vi "Read Field Specs.vi"(8 "error in (no error)":errorcluster, 11 "PitchMessage in":refnum<class "PitchMessage.lvclass">) -> (0 "error out":errorcluster, 2 "Field Specs":T1[](array[typedef])=[{"Name"="Length", "Offset"=0, "Length"=1, "FieldType"=enum."Binary", "FieldValue"=variant}, {"Name"="MessageType", "Offset"=1, "Length"=1, "FieldType"=enum."Value", "FieldValue"=variant}, {"Name"="Time Offset", "Offset"=2, "Length"=4, "FieldType"=enum."Binary", "FieldValue"=variant}, {"Name"="Order Id", "Offset"=6, "Length"=8, "FieldType"=enum."Binary", "FieldValue"=variant}, {"Name"="Side Indicator", "Offset"=14, "Length"=1, "FieldType"=enum."Alphanumeric", "FieldValue"=variant}, {"Name"="Quantity", "Offset"=15, "Length"=4, "FieldType"=enum."Binary", "FieldValue"=variant}, {"Name"="Symbol", "Offset"=19, "Length"=6, "FieldType"=enum."PrintableAscii", "FieldValue"=variant}, {"Name"="Price", "Offset"=25, "Length"=8, "FieldType"=enum."BinaryLongPrice", "FieldValue"=variant}, {"Name"="Add Flags", "Offset"=33, "Length"=1, "FieldType"=enum."BitField", "FieldValue"=variant}], 3 "PitchMessage out":refnum<class "PitchMessage.lvclass">)   [LabVIEW 2020, in "PitchMessage.lvclass"]
uses:
  PitchMessage.lvclass
  FieldSpec.ctl
  PitchMessage.lvclass/PitchMessage.ctl
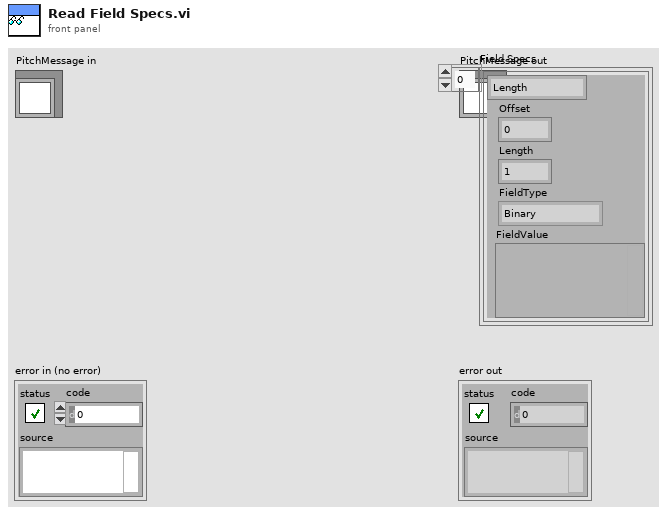
[diagram p1: front panel]
types:
  T1 = typedef "FieldSpec.ctl" = cluster{"Name":string, "Offset":i32, "Length":i32, "FieldType":enum16{"Alphanumeric", "Binary", "BinaryLongPrice", "BinaryShortPrice", "BitField", "PrintableAscii", "Value"}, "FieldValue":variant}
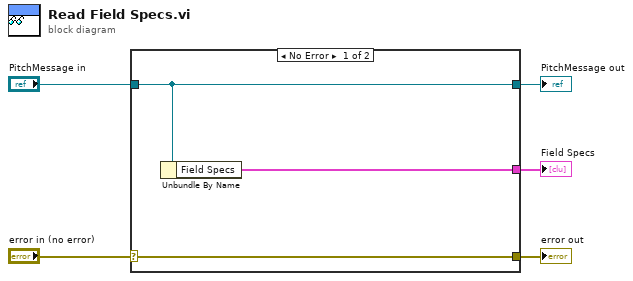
[diagram p0: block diagram]
diagram:
  n1 = case shown="No Error" "error in (no error)" {
    selector: "error in (no error)" -> [w8 w9]
    tunnel: [w8 w9] -> w4
    tunnel: [w7 w10] -> w2
    tunnel: "PitchMessage in" -> [w7 w10]
    tunnel: [w6 _] -> w1
    frame No Error {
      n2 = Unbundle By Name(w7) -> ("Field Specs"=w6:T1[])
    }
    frame Error {
    }
  }
  "error out" <- w4
  "PitchMessage out" <- w2
  "Field Specs" <- w1
